vi "getState.vi"(8 "error in (no error)":errorcluster, 11 "ReadingState in":refnum<class "ManualReadingState.lvclass">) -> (0 "error out":errorcluster, 2 "State":T1=enum."Configuring", 3 "ReadingState out":refnum<class "ManualReadingState.lvclass">)   [LabVIEW 2016, in "ManualReadingState.lvclass"]
uses:
  ManualReadingState.lvclass
  internalState.ctl
  Electrometer.lvclass
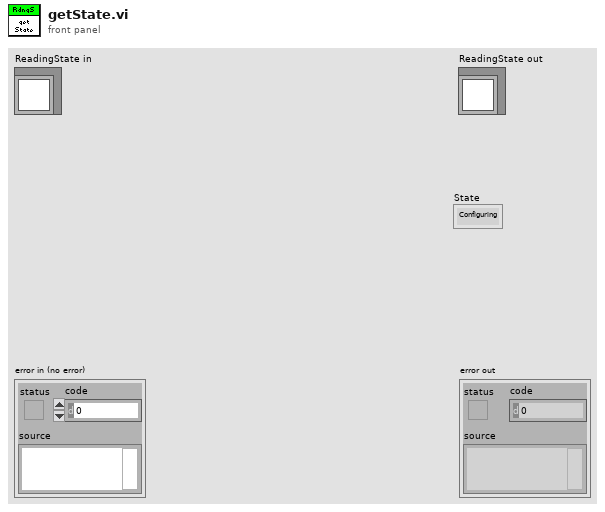
[diagram p1: front panel]
types:
  T1 = typedef "Electrometer.lvclass/internalState.ctl" = enum16{"Ready", "Configuring", "ManualReading", "UntilIntensityReading", "SetDurationReading"}
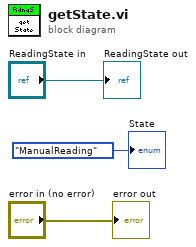
[diagram p0: block diagram]
diagram:
  "error out" <- "error in (no error)"
  "ReadingState out" <- "ReadingState in"
  "State" <- internalState."ManualReading" ("States")
